vi "Channels to plot smart update.vi"(6 "Disable size comparison":bool, 9 "Disable y for 1st channel":bool, 10 "Channels to plot new value":T1[](array[typedef])=[{"Name"="Time", "x"=TRUE, "y"=FALSE}, {"Name"="CH0", "x"=FALSE, "y"=TRUE}], 11 "Channels to plot old value":T1[](array[typedef])=[{"Name"="Time", "x"=TRUE, "y"=FALSE}, {"Name"="CH0", "x"=FALSE, "y"=TRUE}]) -> (3 "Channels to plot out":T1[](array[typedef])=[{"Name"="Time", "x"=TRUE, "y"=FALSE}, {"Name"="CH0", "x"=FALSE, "y"=TRUE}], 5 "Replot?":bool)   [LabVIEW 2015]
uses:
  File/Controls/Channel name entry.ctl
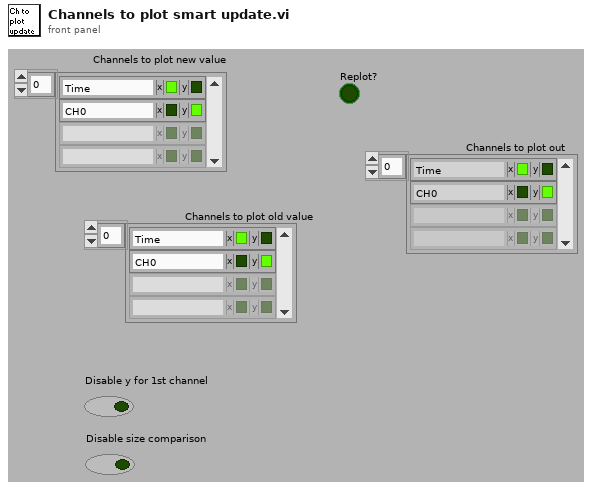
[diagram p1: front panel]
types:
  T1 = typedef "Channel name entry.ctl" = cluster{"Name":string, "x":bool, "y":bool}
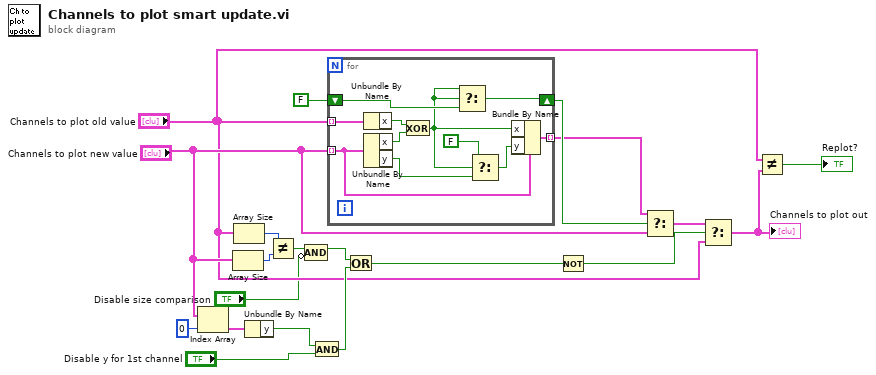
[diagram p0: block diagram]
diagram:
  n1 = Index Array(array="Channels to plot new value", index=0) -> (element=w13:T1)
  n2 = Array Size(array="Channels to plot new value") -> (size(s)=w16:i32)
  n3 = Array Size(array="Channels to plot old value") -> (size(s)=w15:i32)
  n4 = Unbundle By Name(w13) -> ("y"=w8:bool)
  n5 = Not Equal?(x=w15, y=w16) -> (x != y?=w10:bool)
  n6 = Compound Arithmetic op=AND(w10, invert "Disable size comparison") -> (w2:bool)
  n7 = And(x=w8, y="Disable y for 1st channel") -> (x .and. y?=w11:bool)
  n8 = for {
    tunnel: "Channels to plot new value" -> [w28] mode=indexing
    tunnel: "Channels to plot old value" -> [w31] mode=indexing
    tunnel: [w27] -> w18 mode=indexing
    shift-right: [w25] -> w19
    shift-left: FALSE -> [w26]
    n9 = Unbundle By Name(w31) -> ("x"=w29:bool)
    n10 = Unbundle By Name(w28) -> ("x"=w30:bool, "y"=w22:bool)
    n11 = Exclusive Or(1:w30, 2:w29) -> (0:w24:bool)
    n12 = Select(t=w24, s=w24, f=w26) -> (s? t:f=w25:bool)
    n13 = Select(t=FALSE ("Y"), s=w24, f=w22) -> (s? t:f=w21:bool)
    n14 = Bundle By Name(cluster=w28, "x"=w24, "y"=w21) -> (w27:T1)
  }
  n15 = Or(x=w2, y=w11) -> (x .or. y?=w9:bool)
  n16 = Not(x=w9) -> (.not. x?=w6:bool)
  n17 = Select(t=w18, s=w19, f="Channels to plot new value") -> (s? t:f=w17:T1[])
  n18 = Select(t=w17, s=w6, f="Channels to plot old value") -> (s? t:f=w4:T1[])
  "Channels to plot out" <- w4
  n19 = Not Equal?(x="Channels to plot old value", y=w4) -> (x != y?=→"Replot?":bool)
